vi "init_com.vi"(6 "timeout (10sec)":u32=10000, 8 "error in (no error)":errorcluster, 10 "port":u32, 11 "IP address":refnum<visa-resource-name>="COM13") -> (0 "error out":errorcluster)   [LabVIEW 2023, in "BT-Android_interface.lvlib"]
uses:
  BT-Android_interface.lvlib
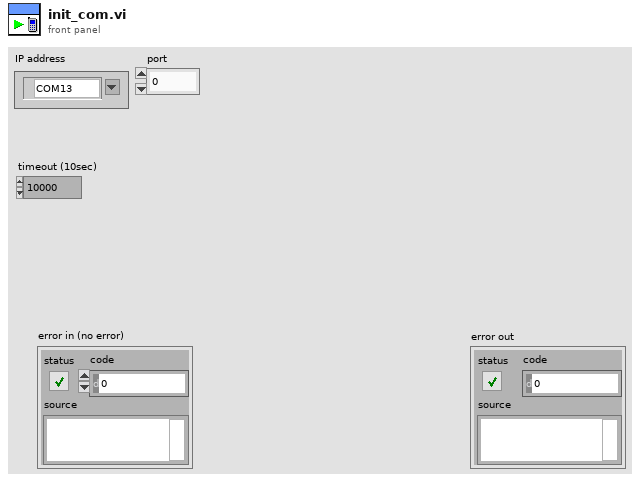
[diagram p1: front panel]
types:
  T1 = enum16{"init", "broadcast_data", "receive_data", "close", "clear_visa"}
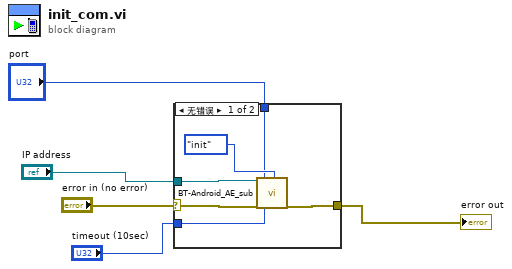
[diagram p0: block diagram]
diagram:
  n1 = case shown="无错误" "error in (no error)" {
    selector: "error in (no error)" -> [w11 w12]
    tunnel: [w10 w12] -> w4
    tunnel: "IP address" -> [w9 _]
    tunnel: "timeout (10sec)" -> [w8 _]
    tunnel: "port" -> [w6 _]
    frame No Error {
      n2 = call "BT-Android_AE_sub.vi"("IP address"=w9, "error in (no error)"=w11, "port"=w6, "timeout (10sec)"=w8, "mode"=T1."init") -> ("error IO"=w10:errorcluster)  [unwired: 13 in, 1 out]
    }
    frame Error {
    }
  }
  "error out" <- w4
